vi "ParseError.vi"(8 "error in (no error)":errorcluster) -> (0 "error out":errorcluster)   [LabVIEW 2020, in "Aerotech.lvlib"]
uses:
  Aerotech.lvlib
  <vilib>/regexp/Match Regular Expression.xnode
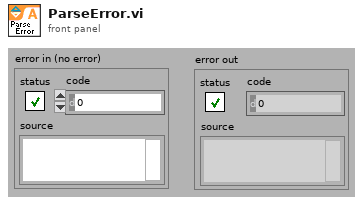
[diagram p1: front panel]
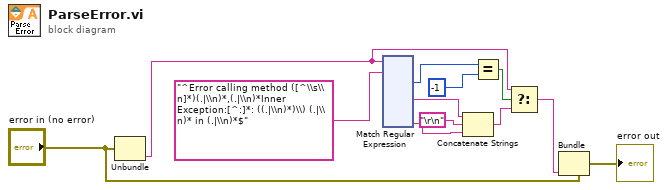
[diagram p0: block diagram]
diagram:
  n1 = Unbundle("error in (no error)") -> ("source"=w4:string)  [unwired: 2 out]
  n2 = xnode "Match Regular Expression"("input string"=w4, "regular expression"="^Error calling method ([^\\s\\n]*)(.|\\n)*,(.|\\n)*Inner Exception:[^:]*: ((.|\\n)*)\\) (.|\\n)* in (.|\\n)*$") -> ("offset past match"=w7:i32, "submatch 1"=w11:string, "submatch 4"=w1:string)  [unwired: 4 in, 6 out]
  n3 = Concatenate Strings(w11, "\r\n", w1) -> (w2:string)
  n4 = Equal?(x=w7, y=-1) -> (x = y?=w5:bool)
  n5 = Select(t=w4, s=w5, f=w2) -> (s? t:f=w3:string)
  n6 = Bundle(cluster="error in (no error)", "source"=w3) -> (→"error out":errorcluster)  [unwired: 2 in]
